vi "Attenuator_CalculatePusle.vi"(0 "计算状态":enum32{"位置-脉冲", "脉冲-位置"}(radio), 1 "数据":dbl) -> (3 "dataout":dbl)   [LabVIEW 2018]
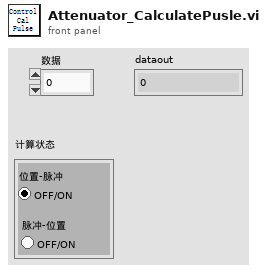
[diagram p1: front panel]
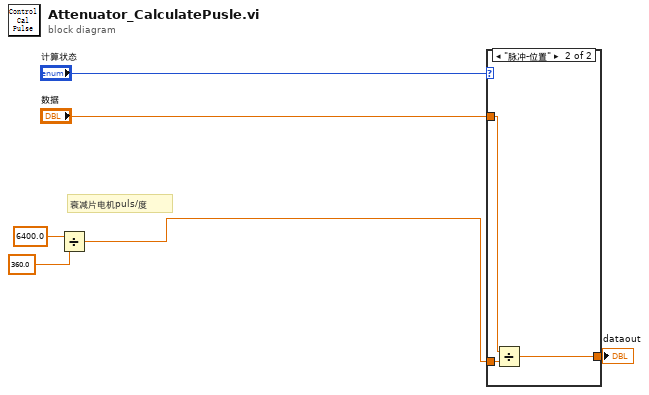
[diagram p0: block diagram]
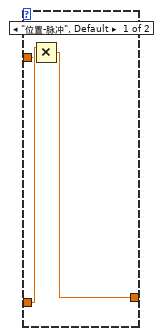
[diagram p2: hidden frame]
diagram:
  # "衰减片电机puls/度"
  n1 = Divide(x=6400.0, y=360.0) -> (x/y=w1:dbl)
  n2 = case shown="\"脉冲-位置\"" "计算状态" {
    tunnel: w1 -> [w9 w10]
    tunnel: [w7 w12] -> w5
    tunnel: "数据" -> [w8 w11]
    frame "位置-脉冲", Default {
      n3 = Multiply(x=w9, y=w8) -> (x*y=w7:dbl)
    }
    frame "脉冲-位置" {
      n4 = Divide(x=w11, y=w10) -> (x/y=w12:dbl)
    }
  }
  "dataout" <- w5
